vi "DjtgSetSpeed.vi"(8 "Error In":errorcluster, 10 "Target Speed (Hz)":u32, 11 "Device Number":u32) -> (0 "Error Out":errorcluster, 2 "Actual JTAG Speed (Hz)":u32, 3 "Device Number":u32)   [LabVIEW 2011, in "LVH-Adept.lvlib" / "DJTG.lvlib"]
doc: "This function is used to set the clock frequency at which TCK will be clocked when shifting data into the JTAG scan chain. The TCK clock frequency will be set to the highest supported value that doesn’t exceed frqReq, or the lowest frequency supported if frqReq is lower than the lowest supported value. The actual clock frequency obtained is returned in frqSet. This function is not supported unless the dprpJtgSetSpeed bit is set in the port properties for the port.\n\nThe clock frequency set will be the highest frequency that will appear on the TCK pin of the port. Depending on the device and the communications protocol used to communicate with the device, the average clock frequency (and therefore the average data rate in to or out of the device) may be lower."
uses:
  DJTG.lvlib
  Private/Type Defs/Error.ctl
  Resources/djtg.dll
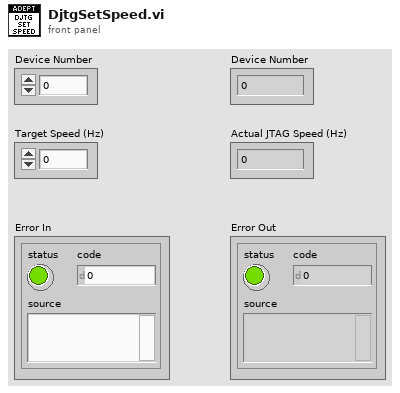
[diagram p1: front panel]
types:
  T1 = typedef "LVH-Adept.lvlib/DJTG.lvlib/Error.ctl" = enum16{"Unknown", "Enable", "PutTmsTdiBits", "GetTdoBits", "Disable", "Close", "Set Aux Reset", "Port Properties", "Get Speed", "Set Speed", "Get Port Count", "Get Batch Properties", "Enable Port", "Set Tmd Tdi Tck", "Get Tms Tdi Tdo Tck", "Put Tdi Bits", "Put Tms Bits", "Clock Tck", "Wait", "Batch", "Flash FPGA"}
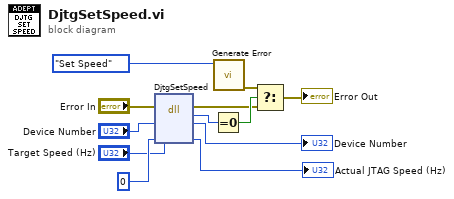
[diagram p0: block diagram]
diagram:
  n1 = dll-call lib="C:/github/labviewhacker/LVH-Adept/LabVIEW/vi.lib/LabVIEW Hacker/Adept/Private/Resources/djtg.dll" fn="DjtgSetSpeed"(error in="Error In", "hif"="Device Number", "frqReq"="Target Speed (Hz)", "pfrqSet"=u32 0 ("pfrqCur")) -> (error out=w7:errorcluster, "Success"=w6:u32, "hif"=→"Device Number":u32, "pfrqSet"=→"Actual JTAG Speed (Hz)":u32)  [unwired: 3 in, 1 out]
  n2 = Equal To 0?(x=w6) -> (x = 0?=w12:bool)
  n3 = call "Generate Error.vi"("DJTG Error"=Error."Set Speed") -> ("Error Out"=w11:errorcluster)  [unwired: 10 in]
  n4 = Select(t=w11, s=w12, f=w7) -> (s? t:f=→"Error Out":errorcluster)
